vi "Pulse Width to Duty Cycle.vi"(1 "frequency":dbl, 2 "pulse width (us)":dbl) -> (0 "duty cycle":dbl)   [LabVIEW 2020]
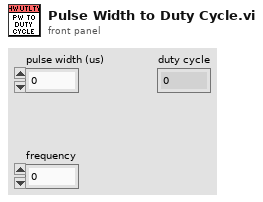
[diagram p1: front panel]
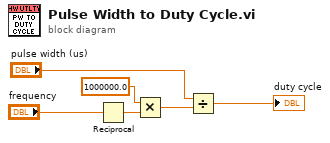
[diagram p0: block diagram]
diagram:
  n1 = Reciprocal(x="frequency") -> (1/x=w4:dbl)
  n2 = Multiply(x=1000000.0, y=w4) -> (x*y=w1:dbl)
  n3 = Divide(x="pulse width (us)", y=w1) -> (x/y=→"duty cycle":dbl)
